vi "getData.vi"(8 "error in (no error)":errorcluster, 10 "Game":refnum<class "Game.lvclass">, 11 "Communication in":refnum<class "Communication.lvclass">) -> (0 "error out":errorcluster, 1 "Total Delay":dbl format="%#.5g", 2 "Robot Data":T1[](array[typedef]), 3 "Communication out":refnum<class "Communication.lvclass">, 4 "Team Color":enum16{"Azul", "Amarelo"}(ring), 5 "AllyRef":refnum<class "Ally.lvclass">)   [LabVIEW 2023, in "Communication.lvclass"]
uses:
  Communication.lvclass
  Game_class/Game.lvclass
  Paths/Convert AI Robot to Robot Command Folder/grSim/grSim Robot Command.ctl
  Ally_class/Ally.lvclass
  Game_class/Game.lvclass/Game.ctl
  Team_class/Team.lvclass/Team.ctl
  Parameters_class/Parameters.lvclass/Parameters.ctl
  Robot_class/Robot.lvclass/Robot.ctl
  Robot_class/Read id.vi
  Robot_class/Read kick_x.vi
  Robot_class/Read kick_z.vi
  Robot_class/Read v_tang.vi
  Robot_class/Read v_norm.vi
  Robot_class/Read v_ang.vi
  Robot_class/Read dribble.vi
  Game_class/Read AllyRef.vi
  Game_class/Read TimeRef.vi
  Game_class/Read KeeperTeam.vi
  Game_class/Read OffensiveTeam.vi
  Game_class/Read DefensiveTeam.vi
  Game_class/Read NavigationTeam.vi
  Game_class/Read Parameters.lvclass.vi
  Parameters_class/Read InvertKick.vi
  Team_class/Read RobotRef.vi
  Team_class/Write RobotRef.vi
  Parameters_class/Parameters.lvclass
  Robot_class/Robot.lvclass
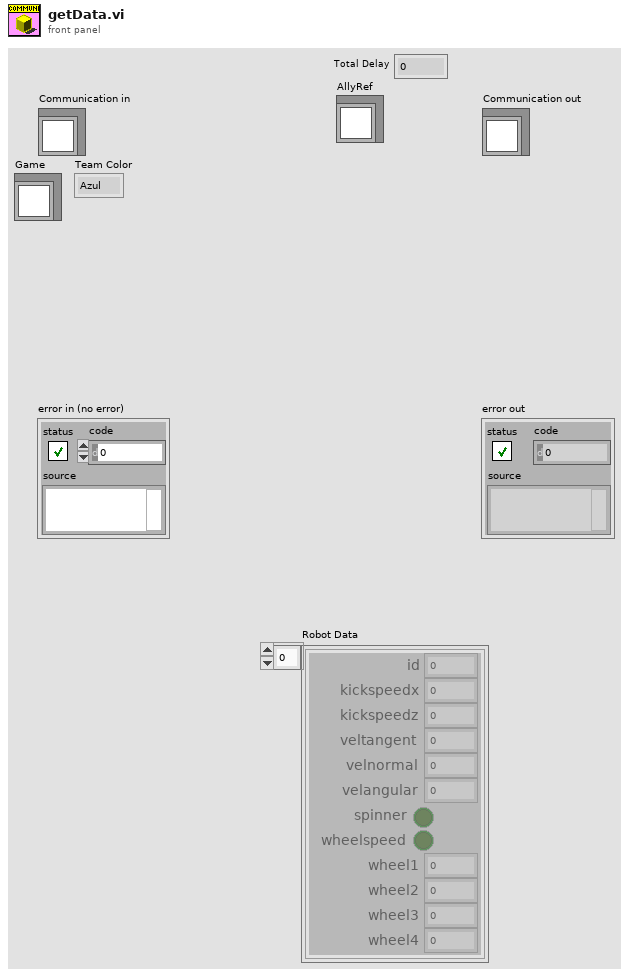
[diagram p1: front panel]
types:
  T1 = typedef "grSim Robot Command.ctl" = cluster{"id":u32, "kickspeedx":sgl, "kickspeedz":sgl, "veltangent":sgl, "velnormal":sgl, "velangular":sgl, "spinner":bool, "wheelspeed":bool, "wheel1":sgl, "wheel2":sgl, "wheel3":sgl, "wheel4":sgl}
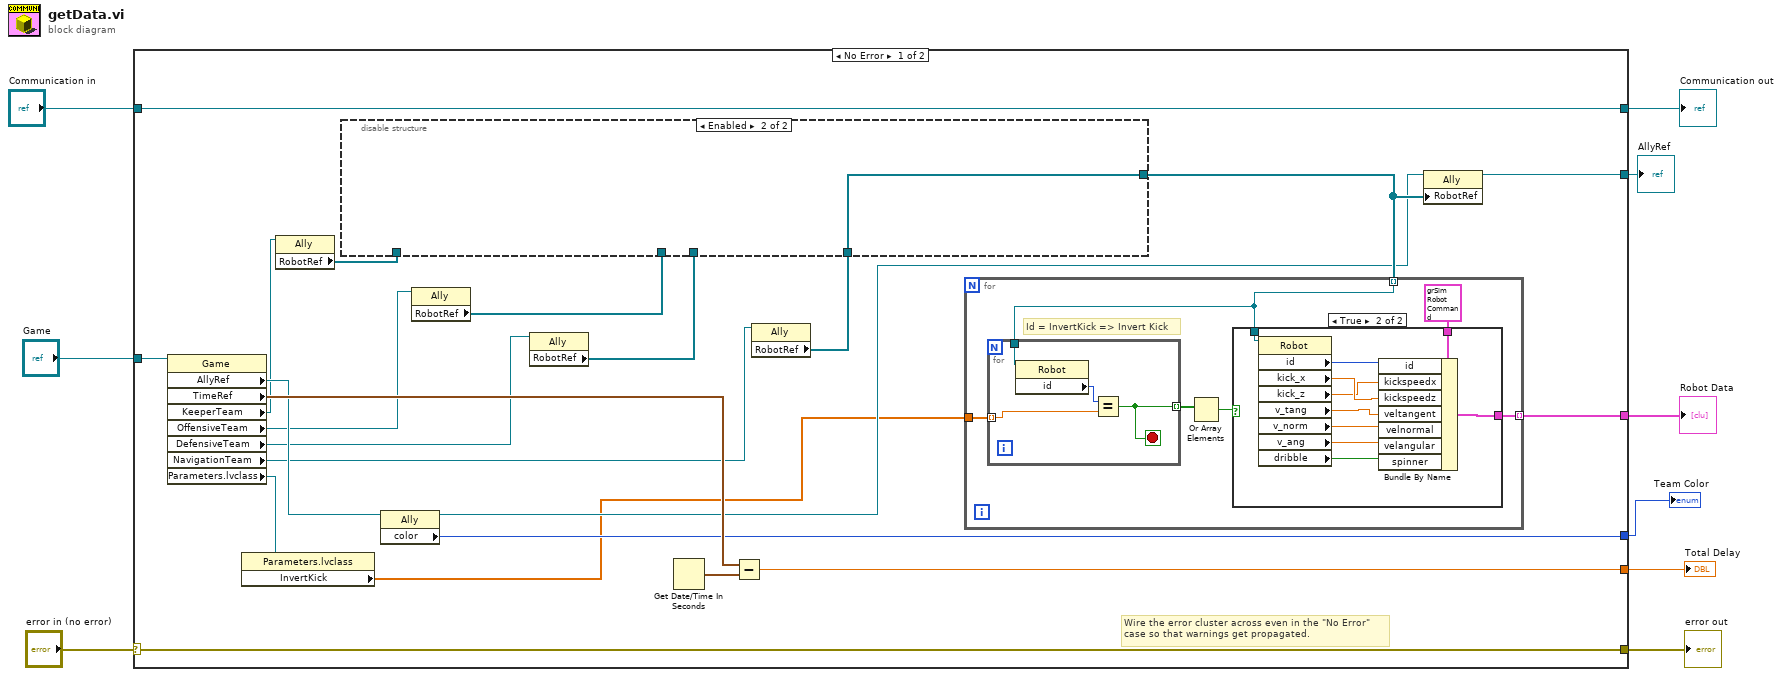
[diagram p0: block diagram]
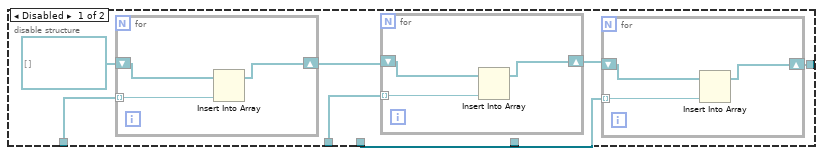
[diagram p2: hidden frame]
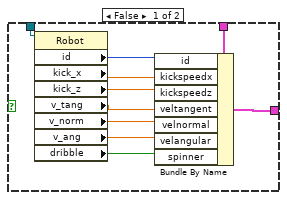
[diagram p3: hidden frame]
diagram:
  n1 = case shown="No Error" "error in (no error)" {
    selector: "error in (no error)" -> [w30 w80]
    tunnel: [w30 w80] -> w8
    tunnel: [w31 w79] -> w6
    tunnel: "Communication in" -> [w31 w79]
    tunnel: "Game" -> [w29 _]
    tunnel: [w27 _] -> w4
    tunnel: [w24 _] -> w3
    tunnel: [w23 _] -> w2
    tunnel: [w15 _] -> w1
    frame No Error {
      # "Wire the error cluster across even in the \"No Error\"\ncase so that warnings get propagated."
      n2 = property class="Game"(reference=w29) -> ("AllyRef"=w25:refnum<class "Ally.lvclass">, "TimeRef"=w28:timestamp, "KeeperTeam"=w22:refnum<class "Ally.lvclass">, "OffensiveTeam"=w20:refnum<class "Ally.lvclass">, "DefensiveTeam"=w18:refnum<class "Ally.lvclass">, "NavigationTeam"=w13:refnum<class "Ally.lvclass">, "Parameters.lvclass"=w11:refnum<class "Parameters.lvclass">)  [unwired: 1 in, 2 out]
      n3 = property class="Parameters.lvclass"(reference=w11) -> ("InvertKick"=w10:dbl[])  [unwired: 1 in, 2 out]
      n4 = property class="Ally"(reference=w22) -> ("RobotRef"=w21:refnum<class "Robot.lvclass">[])  [unwired: 1 in, 2 out]
      n5 = property class="Ally"(reference=w25) -> (reference out=w14:refnum<class "Ally.lvclass">, "color"=w23:enum16{"Azul", "Amarelo"})  [unwired: 1 in, 1 out]
      n6 = property class="Ally"(reference=w20) -> ("RobotRef"=w19:refnum<class "Robot.lvclass">[])  [unwired: 1 in, 2 out]
      n7 = property class="Ally"(reference=w18) -> ("RobotRef"=w17:refnum<class "Robot.lvclass">[])  [unwired: 1 in, 2 out]
      n8 = Get Date/Time In Seconds() -> (seconds since 1Jan1904=w26:timestamp)
      n9 = Subtract(x=w28, y=w26) -> (x-y=w27:dbl)
      n10 = property class="Ally"(reference=w13) -> ("RobotRef"=w12:refnum<class "Robot.lvclass">[])  [unwired: 1 in, 2 out]
      n11 = disable-structure shown="Enabled" {
        disable-tunnel: w21 -> [w38 _]
        disable-tunnel: w19 -> [w36 _]
        disable-tunnel: w17 -> [w33 _]
        disable-tunnel: [w32 w48] -> w16
        disable-tunnel: w12 -> [_ w48]
        frame Disabled {
          n12 = for {
            tunnel: w38 -> [w45] mode=indexing
            shift-right: [w47] -> w35
            shift-left: refnum<class "Robot.lvclass">[] [] -> [w46]
            n13 = Insert Into Array(array=w46, new element=w45) -> (w47:refnum<class "Robot.lvclass">[])  [unwired: 1 in]
          }
          n14 = for {
            tunnel: w36 -> [w42] mode=indexing
            shift-right: [w44] -> w34
            shift-left: w35 -> [w43]
            n15 = Insert Into Array(array=w43, new element=w42) -> (w44:refnum<class "Robot.lvclass">[])  [unwired: 1 in]
          }
          n16 = for {
            tunnel: w33 -> [w39] mode=indexing
            shift-right: [w41] -> w32
            shift-left: w34 -> [w40]
            n17 = Insert Into Array(array=w40, new element=w39) -> (w41:refnum<class "Robot.lvclass">[])  [unwired: 1 in]
          }
        }
        frame Enabled {
        }
      }
      n18 = for {
        tunnel: [w53] -> w24 mode=indexing
        tunnel: w16 -> [w51] mode=indexing
        tunnel: w10 -> [w52]
        # "Id = InvertKick => Invert Kick"
        n19 = for {
          tunnel: w52 -> [w56] mode=indexing
          tunnel: w51 -> [w58]
          tunnel: [w55] -> w49 mode=indexing
          stop <- w55 stop-if-true
          n20 = property class="Robot"(reference=w58) -> ("id"=w57:i32)  [unwired: 1 in, 2 out]
          n21 = Equal?(x=w57, y=w56) -> (x = y?=w55:bool)
        }
        n22 = Or Array Elements(Boolean array=w49) -> (logical OR=w50:bool)
        n23 = case shown="True" w50 {
          tunnel: T1 {"id"=0, "kickspeedx"=0.0, "kickspeedz"=0.0, "veltangent"=0.0, "velnormal"=0.0, "velangular"=0.0, "spinner"=FALSE, "wheelspeed"=FALSE, "wheel1"=0.0, "wheel2"=0.0, "wheel3"=0.0, "wheel4"=0.0} ("grSim Robot Command") -> [w68 w78]
          tunnel: [w61 w73] -> w53
          tunnel: w51 -> [w60 w72]
          frame False {
            n24 = property class="Robot"(reference=w60) -> ("id"=w67:i32, "kick_x"=w66:dbl, "kick_z"=w65:dbl, "v_tang"=w59:dbl, "v_norm"=w64:dbl, "v_ang"=w63:dbl, "dribble"=w62:bool)  [unwired: 1 in, 2 out]
            n25 = Bundle By Name(cluster=w68, "id"=w67, "kickspeedx"=w66, "kickspeedz"=w65, "veltangent"=w59, "velnormal"=w64, "velangular"=w63, "spinner"=w62) -> (w61:T1)
          }
          frame True {
            n26 = property class="Robot"(reference=w72) -> ("id"=w77:i32, "kick_x"=w71:dbl, "kick_z"=w70:dbl, "v_tang"=w69:dbl, "v_norm"=w76:dbl, "v_ang"=w75:dbl, "dribble"=w74:bool)  [unwired: 1 in, 2 out]
            n27 = Bundle By Name(cluster=w78, "id"=w77, "kickspeedx"=w70, "kickspeedz"=w71, "veltangent"=w69, "velnormal"=w76, "velangular"=w75, "spinner"=w74) -> (w73:T1)
          }
        }
      }
      n28 = property class="Ally"(reference=w14, "RobotRef"=w16) -> (reference out=w15:refnum<class "Ally.lvclass">)  [unwired: 1 in, 1 out]
    }
    frame Error {
    }
  }
  "error out" <- w8
  "Communication out" <- w6
  "Total Delay" <- w4
  "Robot Data" <- w3
  "Team Color" <- w2
  "AllyRef" <- w1
